vi "Trigger at Position.vi"(10 "position":u16, 11 "trigger position":u16) -> (3 "trigger":bool)   [LabVIEW 2015, in "Engine Simulation Toolkit.lvlib"]
doc: "If you place multiple of these on the diagram, instead, open this diagram up and place just the first subVI and then multiple of the 2nd subVIs"
uses:
  Engine Simulation Toolkit.lvlib
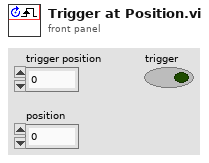
[diagram p1: front panel]
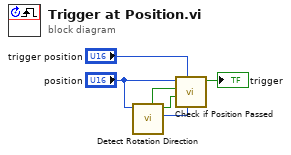
[diagram p0: block diagram]
diagram:
  n1 = call "Detect Rotation Direction.vi"("position"="position") -> ("previous position (n-1)"=w4:u16, "rotated forward or stopped"=w3:bool, "cycle wrapped"=w1:bool)  [unwired: 8 in]
  n2 = call "Check if Position Passed.vi"("previous position (n-1)"=w4, "trigger position"="trigger position", "rotated forward"=w3, "cycle wrapped"=w1, "position"="position") -> ("trigger"=→"trigger":bool)  [unwired: 6 in]
